vi "PostRoom.vi"(8 "error in (no error)":errorcluster, 9 "Data":string, 10 "Enum":T1, 11 "Room Number":i32) -> (0 "error out":errorcluster, 2 "body":string)   [LabVIEW 2015, in "RoomRestApi.lvlib"]
uses:
  RoomRestApi.lvlib
  TypeDef/PostRoomCommands.ctl
  TypeDef/FGVAction.ctl
  <vilib>/httpClient/POSTBuffer.vi
  <vilib>/httpClient/LabVIEWHTTPClient.lvlib
panel:
  out "concatenated string":string
  out "URL":string
  out "headers":string
  # "http://127.0.0.1:8080/RivERWebService/PostRoom?Command={value}&Room={value}"
  # "{\"FlagsState\":\"{\\\"State\\\":[false,false,false,false],\\\"Color\\\":[0,1,2,3]}\"}"
  # "http://127.0.0.1:8001/WebService1/UpdateFlagState?Room={value}&FlagState={value}"
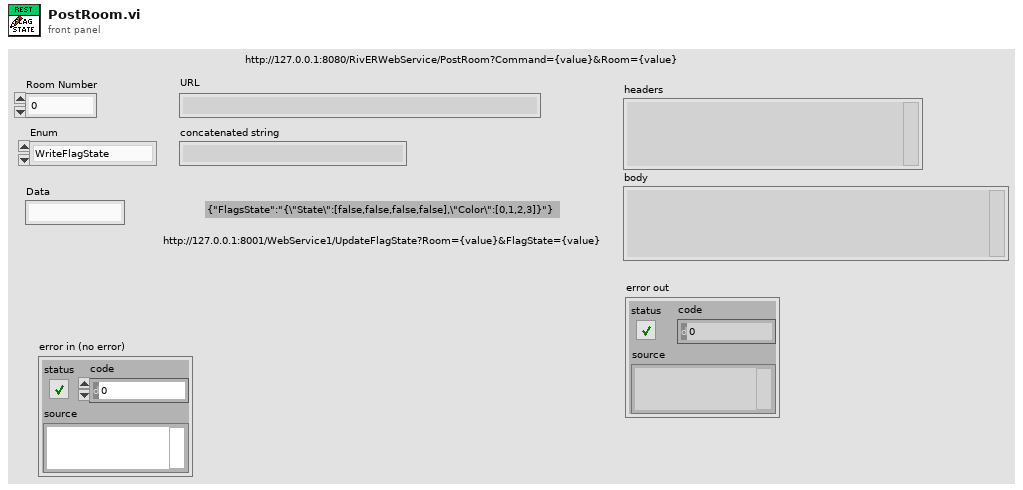
[diagram p1: front panel]
types:
  T1 = typedef "RoomRestApi.lvlib/PostRoomCommands.ctl" = enum16{"WriteFlagState", "WriteFlagColor", "WriteBedVacant", "AddPersonnel", "RemovePersonnel", "AddRequest", "RemoveRequest", "WriteBeaconID", "WriteBedURL", "WriteFlag"}
  T2 = typedef "FGVAction.ctl" = enum16{"Get", "Set"}
  T3 = typedef "LabVIEWHTTPClient.lvlib/ClientHandle.ctl" = refnum<k1>
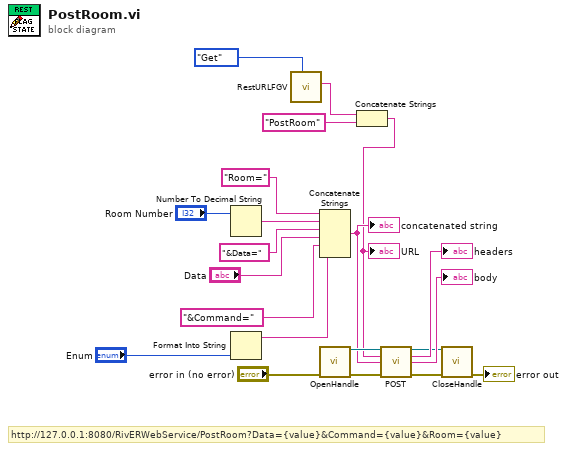
[diagram p0: block diagram]
diagram:
  # "http://127.0.0.1:8080/RivERWebService/PostRoom?Data={value}&Command={value}&Room={value}"
  n1 = Number To Decimal String(number="Room Number") -> (decimal integer string=w11:string)  [unwired: 1 in]
  n2 = Format Into String("Enum") -> (resulting string=w2:string)  [unwired: 3 in, 1 out]
  n3 = call "RestURLFGV.vi"("Action"=FGVAction."Get") -> ("URL"=w7:string)  [unwired: 9 in, 1 out]
  n4 = Concatenate Strings("Room=" ("string"), w11, "&Data=" ("string"), "Data", "&Command=" ("string"), w2) -> (w10:string)
  "concatenated string" <- w10
  n5 = call <vilib>:"OpenHandle.vi"("error in (no error)"="error in (no error)") -> ("client handle out"=w21:T3, "error out"=w16:errorcluster)  [unwired: 13 in]
  n6 = Concatenate Strings(w7, "PostRoom" ("string")) -> (w5:string)
  "URL" <- w5
  n7 = call-poly <vilib>:"POST.vi"("client handle"=w21, "url"=w5, "buffer"=w10, "error in (no error)"=w16) -> ("client handle out"=w18:T3, "headers"=→"headers":string, "body"=→"body":string, "error out"=w17:errorcluster)  [unwired: 8 in]
  n8 = call <vilib>:"CloseHandle.vi"("client handle"=w18, "error in (no error)"=w17) -> ("error out"=→"error out":errorcluster)  [unwired: 13 in]
